vi "large-object-count-parallel-test.vi"(8 "error in (no error)":errorcluster) -> (0 "error out":errorcluster)   [LabVIEW 2013]
uses:
  src/SMO/SMO.lvclass
  <vilib>/addons/_JKI Toolkits/Caraya/classes/Test/Test.lvclass
  <vilib>/addons/_JKI Toolkits/Caraya/classes/Assert/Assert.lvclass
panel:
  in  "Instances":i32=10
  out "Total Time":dbl
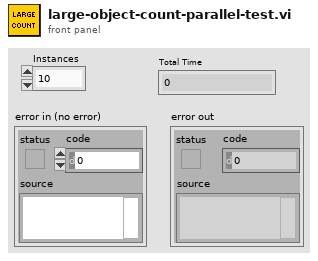
[diagram p1: front panel]
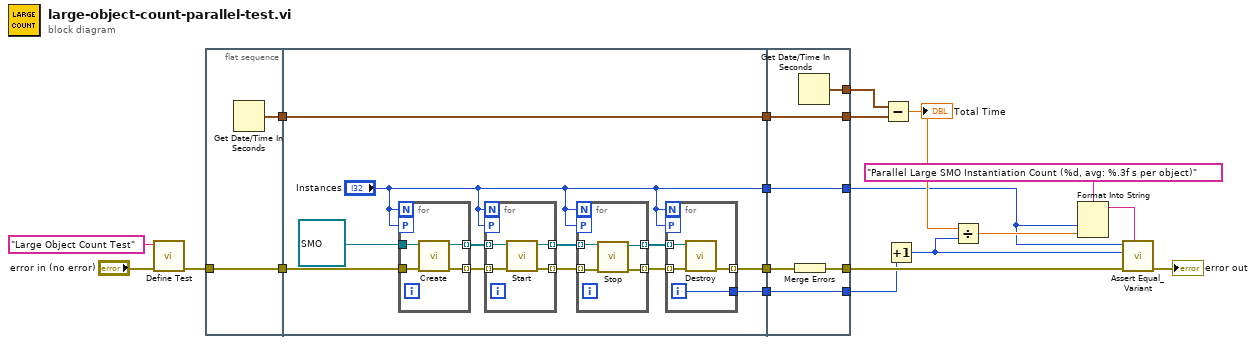
[diagram p0: block diagram]
diagram:
  n1 = call <vilib>:"Define Test.vi"("error in (no error)"="error in (no error)", "Label (VI Title)"="Large Object Count Test") -> ("error out"=w18:errorcluster)  [unwired: 9 in]
  n2 = flat-sequence {
    tunnel: w18 -> [w22]
    tunnel: [w22] -> w9
    tunnel: [w21] -> w4
    tunnel: w9 -> [w33]
    tunnel: [w25] -> w8
    tunnel: ["Instances"] -> w7
    tunnel: [w32] -> w5
    tunnel: w4 -> [w32]
    tunnel: [w24] -> w1
    tunnel: [w55] -> w10
    tunnel: [w52] -> w17
    tunnel: w8 -> [w56]
    tunnel: w7 -> [w55]
    tunnel: [w54] -> w6
    tunnel: w5 -> [w54]
    tunnel: [w53] -> w3
    tunnel: [w51] -> w2
    tunnel: w1 -> [w51]
    frame #0 {
      n3 = Get Date/Time In Seconds() -> (seconds since 1Jan1904=w21:timestamp)
    }
    frame #1 {
      n4 = for {
        N: "Instances" -> [_]
        tunnel: refnum<class "SMO.lvclass"> refnum ("SMO.lvclass") -> [w50]
        tunnel: w33 -> [w49]
        tunnel: [w48] -> w30 mode=indexing
        workers-P: "Instances" -> [_]
        tunnel: [w47] -> w31 mode=indexing
        n5 = call "Create.vi"("error in (no error)"=w49, "SMO"=w50) -> ("error out"=w48:errorcluster, "SMO out"=w47:refnum<class "SMO.lvclass">)  [unwired: 7 in, 1 out]
      }
      n6 = for {
        N: "Instances" -> [_]
        tunnel: w31 -> [w46] mode=indexing
        tunnel: w30 -> [w44] mode=indexing
        tunnel: [w43] -> w28 mode=indexing
        workers-P: "Instances" -> [_]
        tunnel: [w45] -> w29 mode=indexing
        n7 = call "Start.vi"("error in (no error)"=w44, "SMO"=w46) -> ("error out"=w43:errorcluster, "SMO out"=w45:refnum<class "SMO.lvclass">)  [unwired: 8 in]
      }
      n8 = for {
        N: "Instances" -> [_]
        tunnel: w29 -> [w42] mode=indexing
        tunnel: w28 -> [w41] mode=indexing
        tunnel: [w39] -> w26 mode=indexing
        workers-P: "Instances" -> [_]
        tunnel: [w40] -> w27 mode=indexing
        n9 = call "Stop.vi"("error in (no error)"=w41, "SMO"=w42) -> ("error out"=w39:errorcluster, "SMO out"=w40:refnum<class "SMO.lvclass">)  [unwired: 8 in]
      }
      n10 = for {
        N: "Instances" -> [_]
        tunnel: w27 -> [w38] mode=indexing
        tunnel: w26 -> [w37] mode=indexing
        workers-P: "Instances" -> [_]
        tunnel: [w36] -> w25 mode=indexing
        tunnel: [w35] -> w24
        i -> [w35]
        n11 = call "Destroy.vi"("error in (no error)"=w37, "SMO"=w38) -> ("error out"=w36:errorcluster)  [unwired: 9 in]
      }
    }
    frame #2 {
      n12 = Merge Errors(w56) -> (w52:errorcluster)
      n13 = Get Date/Time In Seconds() -> (seconds since 1Jan1904=w53:timestamp)
    }
  }
  n14 = Subtract(x=w3, y=w6) -> (x-y=w15:dbl)
  "Total Time" <- w15
  n15 = Increment(x=w2) -> (x+1=w14:i32)
  n16 = Divide(x=w15, y=w14) -> (x/y=w13:dbl)
  n17 = Format Into String(format string="Parallel Large SMO Instantiation Count (%d, avg: %.3f s per object)" ("Label"), w10, w13) -> (resulting string=w12:string)  [unwired: 2 in, 1 out]
  n18 = call <vilib>:"Assert Equal_Variant.vi"("Label"=w12, "error in (no error)"=w17, "Y"=w14, "X"=w10) -> ("error out"=→"error out":errorcluster)  [unwired: 7 in]
